vi "Main.vi"(11 "_Rescript Msg in":refnum<class "_Msg Rescript.lvclass">) -> (0 "error out":errorcluster, 3 "_Rescript Msg out":refnum<class "_Msg Rescript.lvclass">)   [LabVIEW 2025, in "_Msg Rescript.lvlib" / "_Msg Rescript.lvclass"]
uses:
  _Msg Rescript.lvclass
  _Msg Rescript.lvclass/_Msg Rescript.ctl
  _Shared/Name Specs/Name Specs.lvclass
  _Shared/Project Stuff/Project Stuff.lvclass
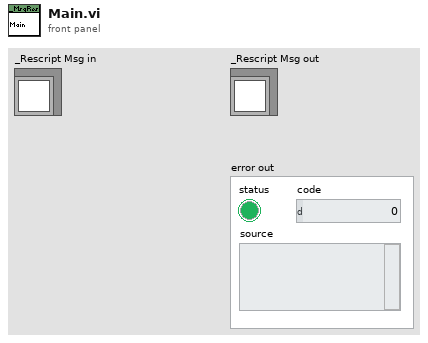
[diagram p1: front panel]
types:
  T1 = typedef "_Shared.lvlib/Name Stuff.ctl" = cluster{"Type (Enum)":T2, "Type (String)":string, "Name Library File Path":path, "Name":string, "Name Type":string}
  T2 = typedef "_Shared.lvlib/Type.ctl" = enum16{"Actor", "Msg"}
  T3 = typedef "_Msg Rescript.lvlib/_Msg Rescript.lvclass/Name Refs.ctl" = cluster{"Name VI":refnum<vi>}
  T4 = typedef "_Msg Rescript.lvlib/_Msg Rescript.lvclass/Name Msg Refs.ctl" = cluster{"Private Data Control":refnum<vi>, "Private Data Cluster":refnum<vi>, "Init Msg VI":refnum<vi>, "Msg VI":refnum<vi>}
  T5 = typedef "_Msg Rescript.lvlib/_Msg Rescript.lvclass/Name Msg Output Refs.ctl" = cluster{"Private Data Control":refnum<vi>, "Private Data Cluster":refnum<vi>, "Init Msg Output VI":refnum<vi>, "Read Msg Output VI":refnum<vi>}
  T6 = typedef "_Msg Rescript.lvlib/_Msg Rescript.lvclass/VI Refs.ctl" = cluster{"Name VI":refnum<vi>, "Call VI":refnum<vi>, "Recurse VI":refnum<vi>, "Tell Self VI":refnum<vi>, "Tell Parent VI":refnum<vi>, "Tell Child VI":refnum<vi>, "Tell Reply VI":refnum<vi>}
  T7 = typedef "_Msg Rescript.lvlib/_Msg Rescript.lvclass/Terminal Attributes.ctl" = map{i32, T8}
  T8 = typedef "_Msg Rescript.lvlib/_Msg Rescript.lvclass/Attributes.ctl" = cluster{"Control":refnum<vi>, "Wire Rule":enum16{"Invalid Wire Rule", "Required", "Recommended", "Optional", "Dynamic Dispatch"}}
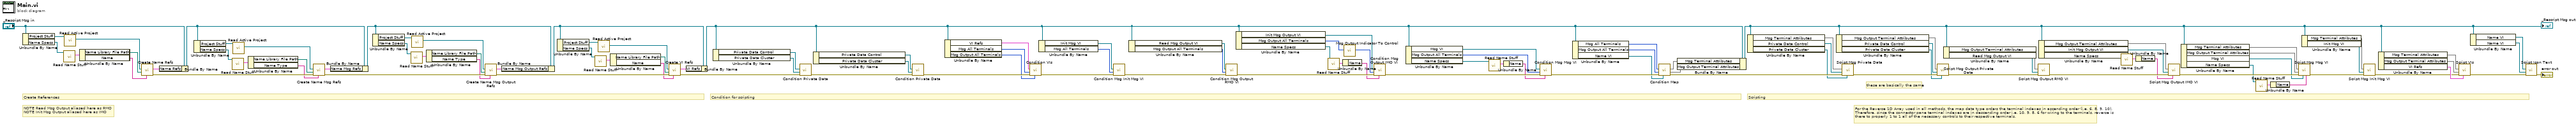
[diagram p0: block diagram]
diagram:
  # "NOTE Read Msg Output aliased here as RMO\nNOTE Init Msg Output aliased here as IMO"
  # "these are basically the same"
  # "these are basically the same"
  # "Create References"
  # "Scripting"
  # "Condition for scripting"
  # "For the Reverse 1D Array used in all methods, the map data type orders the terminal indexes in ascending order (i.e. 6, 8, 9, 10). Therefore, since the connector pane terminal indexes are in descending order i.e. 10, 9, 8, 6 for wiring to the terminals, reverse is there to properly 1 to 1 all of the necessary controls to their respective terminals."
  n1 = Unbundle By Name("_Rescript Msg in") -> ("Project Stuff"=w12:refnum<class "Project Stuff.lvclass">, "Name Specs"=w88:refnum<class "Name Specs.lvclass">)
  n2 = call "Read Name Stuff.vi"("Name Specs in"=w88) -> ("Name Stuff"=w87:T1)  [unwired: 10 in]
  n3 = call "Read Active Project.vi"("Project Stuff in"=w12) -> ("Active Project"=w11:refnum<vi>)  [unwired: 10 in]
  n4 = Unbundle By Name(w87) -> ("Name Library File Path"=w14:path, "Name"=w13:string)
  n5 = call "Create Name Refs.vi"("Name"=w13, "Name Library File Path"=w14, "Active Project"=w11) -> ("error out"=w93:errorcluster, "Name Refs"=w86:T3)  [unwired: 7 in]
  n6 = Bundle By Name(cluster="_Rescript Msg in", "Name Refs"=w86) -> (w83:refnum<class "_Msg Rescript.lvclass">)
  n7 = Unbundle By Name(w83) -> ("Project Stuff"=w82:refnum<class "Project Stuff.lvclass">, "Name Specs"=w84:refnum<class "Name Specs.lvclass">)
  n8 = call "Read Name Stuff.vi"("Name Specs in"=w84) -> ("Name Stuff"=w85:T1)  [unwired: 10 in]
  n9 = call "Read Active Project.vi"("Project Stuff in"=w82) -> ("Active Project"=w81:refnum<vi>)  [unwired: 10 in]
  n10 = Unbundle By Name(w85) -> ("Name Library File Path"=w80:path, "Name Type"=w79:string)
  n11 = call "Create Name Msg Refs.vi"("Name Msg"=w79, "error in"=w93, "Name Library File Path"=w80, "Active Project"=w81) -> ("error out"=w92:errorcluster, "Name Msg Refs"=w78:T4)  [unwired: 6 in]
  n12 = Bundle By Name(cluster=w83, "Name Msg Refs"=w78) -> (w74:refnum<class "_Msg Rescript.lvclass">)
  n13 = Unbundle By Name(w74) -> ("Project Stuff"=w77:refnum<class "Project Stuff.lvclass">, "Name Specs"=w76:refnum<class "Name Specs.lvclass">)
  n14 = call "Read Name Stuff.vi"("Name Specs in"=w76) -> ("Name Stuff"=w75:T1)  [unwired: 10 in]
  n15 = call "Read Active Project.vi"("Project Stuff in"=w77) -> ("Active Project"=w73:refnum<vi>)  [unwired: 10 in]
  n16 = Unbundle By Name(w75) -> ("Name Library File Path"=w72:path, "Name Type"=w71:string)
  n17 = call "Create Name Msg Output Refs.vi"("Name Msg"=w71, "error in"=w92, "Name Library File Path"=w72, "Active Project"=w73) -> ("error out"=w91:errorcluster, "Name Msg Output Refs"=w70:T5)  [unwired: 6 in]
  n18 = Bundle By Name(cluster=w74, "Name Msg Output Refs"=w70) -> (w67:refnum<class "_Msg Rescript.lvclass">)
  n19 = Unbundle By Name(w67) -> ("Project Stuff"=w10:refnum<class "Project Stuff.lvclass">, "Name Specs"=w69:refnum<class "Name Specs.lvclass">)
  n20 = call "Read Name Stuff.vi"("Name Specs in"=w69) -> ("Name Stuff"=w68:T1)  [unwired: 10 in]
  n21 = call "Read Active Project.vi"("Project Stuff in"=w10) -> ("Active Project"=w7:refnum<vi>)  [unwired: 10 in]
  n22 = Unbundle By Name(w68) -> ("Name Library File Path"=w8:path, "Name"=w9:string)
  n23 = call "Create VI Refs.vi"("Name"=w9, "error in"=w91, "Name Library File Path"=w8, "Active Project"=w7) -> ("error out"=w90:errorcluster, "VI Refs"=w66:T6)  [unwired: 6 in]
  n24 = Bundle By Name(cluster=w67, "VI Refs"=w66) -> (w56:refnum<class "_Msg Rescript.lvclass">)
  n25 = Unbundle By Name(w56) -> ("Private Data Control"=w101:refnum<vi>, "Private Data Cluster"=w100:refnum<vi>)
  n26 = call "Condition Private Data.vi"("error in"=w90, "Private Data Cluster"=w100, "Private Data Control"=w101) -> ("error out"=w65:errorcluster)  [unwired: 8 in]
  n27 = Unbundle By Name(w56) -> ("Private Data Control"=w63:refnum<vi>, "Private Data Cluster"=w62:refnum<vi>)
  n28 = call "Condition Private Data.vi"("error in"=w65, "Private Data Cluster"=w62, "Private Data Control"=w63) -> ("error out"=w64:errorcluster)  [unwired: 8 in]
  n29 = Unbundle By Name(w56) -> ("VI Refs"=w95:T6, "Msg All Terminals"=w61:i32[], "Msg Output All Terminals"=w57:i32[])
  n30 = call "Condition VIs.vi"("Msg Output All Terminals"=w57, "error in"=w64, "Msg All Terminals"=w61, "VI Refs"=w95) -> ("error out"=w96:errorcluster)  [unwired: 7 in]
  n31 = Unbundle By Name(w56) -> ("Init Msg VI"=w98:refnum<vi>, "Msg All Terminals"=w97:i32[])
  n32 = call "Condition Msg Init Msg VI.vi"("error in"=w96, "Msg All Terminals"=w97, "Name Msg Refs.Init Msg VI"=w98) -> ("error out"=w60:errorcluster)  [unwired: 8 in]
  n33 = Unbundle By Name(w56) -> ("Read Msg Output VI"=w55:refnum<vi>, "Msg Output All Terminals"=w54:i32[])
  n34 = call "Condition Msg Output RMO VI.vi"("error in"=w60, "Msg Output All Terminals"=w54, "Name Msg Output Refs.Read Msg Output VI"=w55) -> ("error out"=w59:errorcluster)  [unwired: 8 in]
  n35 = Unbundle By Name(w56) -> ("Init Msg Output VI"=w53:refnum<vi>, "Msg Output All Terminals"=w2:i32[], "Name Specs"=w52:refnum<class "Name Specs.lvclass">)
  n36 = call "Read Name Stuff.vi"("Name Specs in"=w52) -> ("Name Stuff"=w51:T1)  [unwired: 10 in]
  n37 = Unbundle By Name(w51) -> ("Name"=w50:string)
  n38 = call "Msg Output Indicator To Control.vi"("Msg Output All Terminals"=w2) -> ("Msg Output All Terminals (For Init Msg Output.vi)"=w1:i32[])  [unwired: 10 in]
  n39 = call "Condition Msg Output IMO VI.vi"("Name"=w50, "error in"=w59, "Msg Output All Terminals (For Init Msg Output.vi)"=w1, "Name Msg Output Refs.Init Msg Output VI"=w53) -> ("error out"=w58:errorcluster)  [unwired: 7 in]
  n40 = Unbundle By Name(w56) -> ("Msg VI"=w99:refnum<vi>, "Msg Output All Terminals"=w3:i32[], "Name Specs"=w5:refnum<class "Name Specs.lvclass">)
  n41 = call "Read Name Stuff.vi"("Name Specs in"=w5) -> ("Name Stuff"=w6:T1)  [unwired: 10 in]
  n42 = Unbundle By Name(w6) -> ("Name"=w4:string)
  n43 = call "Condition Msg Msg VI.vi"("Name"=w4, "error in"=w58, "Msg Output All Terminals"=w3, "Name Msg Refs.Msg VI"=w99) -> ("error out"=w107:errorcluster)  [unwired: 7 in]
  n44 = Unbundle By Name(w56) -> ("Msg All Terminals"=w45:i32[], "Msg Output All Terminals"=w46:i32[], "Name VI"=w47:refnum<vi>)
  n45 = call "Condition Map.vi"("Name Refs.Name VI"=w47, "error in"=w107, "Msg Output All Terminals"=w46, "Msg All Terminals"=w45) -> ("error out"=w106:errorcluster, "Msg Output Terminal Attributes"=w48:T7, "Msg Terminal Attributes"=w49:T7)  [unwired: 5 in]
  n46 = Bundle By Name(cluster=w56, "Msg Terminal Attributes"=w49, "Msg Output Terminal Attributes"=w48) -> (w33:refnum<class "_Msg Rescript.lvclass">)
  "_Rescript Msg out" <- w33
  n47 = Unbundle By Name(w33) -> ("Msg Terminal Attributes"=w40:T7, "Private Data Control"=w39:refnum<vi>, "Private Data Cluster"=w38:refnum<vi>)
  n48 = Unbundle By Name(w33) -> ("Msg Output Terminal Attributes"=w37:T7, "Private Data Control"=w36:refnum<vi>, "Private Data Cluster"=w35:refnum<vi>)
  n49 = call "Script Msg Private Data.vi"("Name Msg Refs.Private Data Cluster"=w38, "error in"=w106, "Name Msg Refs.Private Data Control"=w39, "Msg Terminal Attributes"=w40) -> ("error out"=w41:errorcluster)  [unwired: 7 in]
  n50 = call "Script Msg Output Private Data.vi"("Name Msg Output Refs.Private Data Cluster"=w35, "error in"=w41, "Name Msg Output Refs.Private Data Control"=w36, "Msg Output Terminal Attributes"=w37) -> ("error out"=w31:errorcluster)  [unwired: 7 in]
  n51 = Unbundle By Name(w33) -> ("Msg Output Terminal Attributes"=w29:T7, "Read Msg Output VI"=w28:refnum<vi>)
  n52 = call "Script Msg Output RMO VI.vi"("error in"=w31, "Name Msg Output Refs.Read Msg Output VI"=w28, "Msg Output Terminal Attributes"=w29) -> ("error out"=w32:errorcluster)  [unwired: 8 in]
  n53 = Unbundle By Name(w33) -> ("Msg Output Terminal Attributes"=w27:T7, "Init Msg Output VI"=w26:refnum<vi>, "Name Specs"=w24:refnum<class "Name Specs.lvclass">)
  n54 = call "Read Name Stuff.vi"("Name Specs in"=w24) -> ("Name Stuff"=w25:T1)  [unwired: 10 in]
  n55 = Unbundle By Name(w25) -> ("Name"=w23:string)
  n56 = call "Script Msg Output IMO VI.vi"("Name"=w23, "error in"=w32, "Name Msg Output Refs.Init Msg Output VI"=w26, "Msg Output Terminal Attributes"=w27) -> ("error out"=w30:errorcluster)  [unwired: 7 in]
  n57 = Unbundle By Name(w33) -> ("Msg Terminal Attributes"=w17:T7, "Msg Output Terminal Attributes"=w18:T7, "Msg VI"=w20:refnum<vi>, "Name Specs"=w21:refnum<class "Name Specs.lvclass">)
  n58 = call "Read Name Stuff.vi"("Name Specs in"=w21) -> ("Name Stuff"=w22:T1)  [unwired: 10 in]
  n59 = Unbundle By Name(w22) -> ("Name"=w19:string)
  n60 = call "Script Msg Msg VI.vi"("Name"=w19, "Name Msg Refs.Msg VI"=w20, "error in"=w30, "Msg Output Terminal Attributes"=w18, "Msg Terminal Attributes"=w17) -> ("error out"=w94:errorcluster)  [unwired: 6 in]
  n61 = Unbundle By Name(w33) -> ("Msg Terminal Attributes"=w16:T7, "Init Msg VI"=w15:refnum<vi>)
  n62 = call "Script Msg Init Msg VI.vi"("error in"=w94, "Name Msg Refs.Init Msg VI"=w15, "Msg Terminal Attributes"=w16) -> ("error out"=w34:errorcluster)  [unwired: 8 in]
  n63 = Unbundle By Name(w33) -> ("Msg Terminal Attributes"=w44:T7, "Msg Output Terminal Attributes"=w43:T7, "VI Refs"=w42:T6)
  n64 = call "Script VIs.vi"("VI Refs"=w42, "error in"=w34, "Msg Output Terminal Attributes"=w43, "Msg Terminal Attributes"=w44) -> ("error out"=w103:errorcluster)  [unwired: 7 in]
  n65 = Unbundle By Name(w33) -> ("Name VI"=w105:refnum<vi>, "Name VI"=w104:refnum<vi>)
  n66 = call "Script Icon Text.vi"("error in"=w103, "VI Refs.Name VI"=w104, "Name Refs.Name VI"=w105) -> ("error out"=→"error out":errorcluster)  [unwired: 8 in]
